vi "TrapProfile_Execute_AtGoal.vi"(3 "PositionTolerance":dbl=0.05 format="%16.4g", 5 "VelocityTolerance":dbl=9.9e+30 format="%16.4g", 7 "ConsecutiveAtGoalCount":i32=1, 8 "CurrentVelocity":dbl format="%16.4g", 9 "CurrentPosition":dbl format="%16.4g", 10 "GoalVelocity":dbl format="%16.4g", 11 "GoalPosition":dbl format="%16.4g") -> (2 "AtGoal":bool)   [LabVIEW 2019, in "Trajectory_Library.lvlib"]
doc: "Convience function to determine if the trapezoid profile goal has been reached.\n\nInputs:\n - Position Tolerance -- Allowed position tolerance\n - Velocity Tolerance -- Allowed velocity tolerance (Default 9.9E+30)\n - ConsecutiveAtGoalCount -- How many times the position and velocity errors have to be within the tolerance to be considered \"At Goal\"\n - Goal Position -- Deisred final position\n - Goal Velocity -- Desired velocity when goal position is reached. (Might often be zero.)\n - Current Position -- Current position (This could be a measured value.)\n - Current Velocity -- Current velocity (This could be a measured value.)\n\nOutputs:\n - AtGoal -- The position and velocity errors have been within defined tolerance for at least the defined consecutive scan times."
uses:
  Trajectory_Library.lvlib
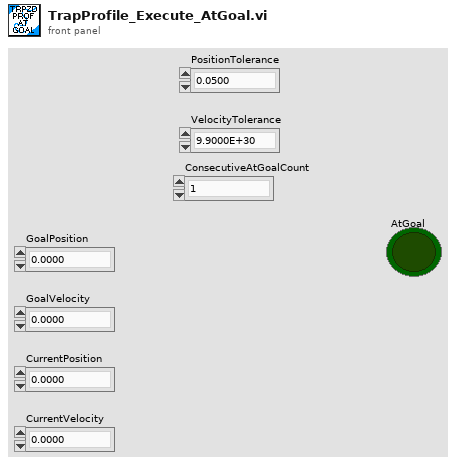
[diagram p1: front panel]
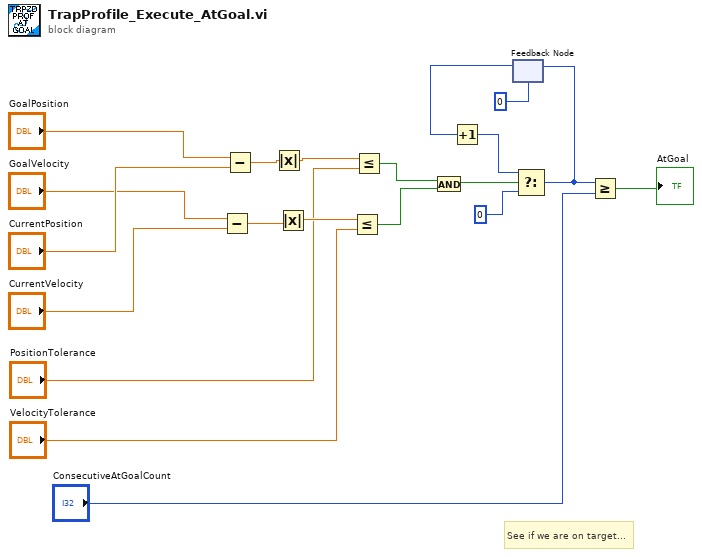
[diagram p0: block diagram]
diagram:
  # "See if we are on target..."
  n1 = Subtract(x="GoalVelocity", y="CurrentVelocity") -> (x-y=w15:dbl)
  n2 = Subtract(x="GoalPosition", y="CurrentPosition") -> (x-y=w16:dbl)
  n3 = Absolute Value(x=w16) -> (abs(x)=w13:dbl)
  n4 = Absolute Value(x=w15) -> (abs(x)=w14:dbl)
  n5 = Less Or Equal?(x=w14, y="VelocityTolerance") -> (x <= y?=w9:bool)
  n6 = Less Or Equal?(x=w13, y="PositionTolerance") -> (x <= y?=w10:bool)
  n7 = And(x=w10, y=w9) -> (x .and. y?=w8:bool)
  n8 = feedback #1(0 ("f")) -> (w6:i32)
  n9 = Increment(x=w6) -> (x+1=w5:i32)
  n10 = Select(t=w5, s=w8, f=0) -> (s? t:f=w3:i32)
  n11 = feedback-in #1(w3) -> ()
  n12 = Greater Or Equal?(x=w3, y="ConsecutiveAtGoalCount") -> (x >= y?=→"AtGoal":bool)
